vi "Segment_g.vi"(11 "Boolean Array":bool[](array[boolean])) -> (3 "Segment g":bool)   [LabVIEW 2024]
panel:
  out "D":bool
  out "C":bool
  out "B":bool
  out "A":bool
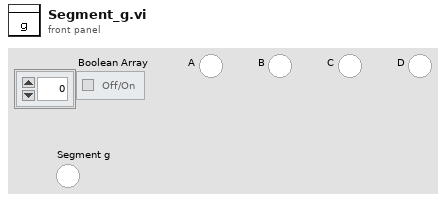
[diagram p1: front panel]
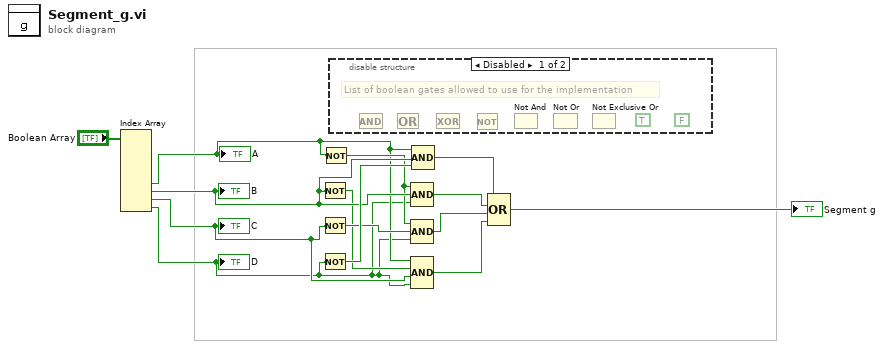
[diagram p0: block diagram]
diagram:
  n1 = Index Array(array="Boolean Array") -> (element #5=w9:bool, element #6=w12:bool, element #7=w7:bool, element #8=w6:bool)  [unwired: 8 in, 4 out]
  "A" <- w9
  "B" <- w12
  "C" <- w7
  "D" <- w6
  n2 = Not(x=w12) -> (.not. x?=w8:bool)
  n3 = Not(x=w7) -> (.not. x?=w10:bool)
  n4 = Not(x=w6) -> (.not. x?=w13:bool)
  n5 = Not(x=w9) -> (.not. x?=w11:bool)
  n6 = disable-structure shown="Disabled" {
    frame Disabled {
      (unwired) FALSE
      (unwired) TRUE
      # "List of boolean gates allowed to use for the implementation"
      n7 = And() -> ()  [unwired: 2 in, 1 out]
      n8 = Or() -> ()  [unwired: 2 in, 1 out]
      n9 = Exclusive Or() -> ()  [unwired: 2 in, 1 out]
      n10 = Not() -> ()  [unwired: 1 in, 1 out]
      n11 = Not And() -> ()  [unwired: 2 in, 1 out]
      n12 = Not Or() -> ()  [unwired: 2 in, 1 out]
      n13 = Not Exclusive Or() -> ()  [unwired: 2 in, 1 out]
    }
    frame Enabled {
    }
  }
  n14 = Compound Arithmetic op=AND(w11, w12, w6) -> (w3:bool)
  n15 = Compound Arithmetic op=AND(w11, w10, w6) -> (w4:bool)
  n16 = Compound Arithmetic op=AND(w9, w8, w7, w6) -> (w5:bool)
  n17 = Compound Arithmetic op=AND(w9, w12, w13) -> (w2:bool)
  n18 = Compound Arithmetic op=OR(w2, w3, w4, w5) -> (→"Segment g":bool)
